vi "Clear.vi"(8 "error in (no error)":errorcluster, 11 "Execution UI In":refnum<class "Execution UI.lvclass">) -> (0 "error out":errorcluster)   [LabVIEW 2020, in "Execution UI.lvclass"]
uses:
  Execution UI.lvclass
  Execution UI.lvclass/Execution UI.ctl
  Process/Process.lvclass
  Result Model/Result Model.lvclass
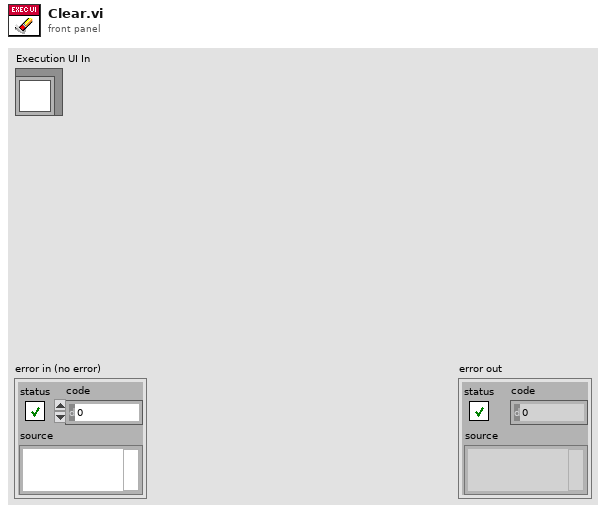
[diagram p1: front panel]
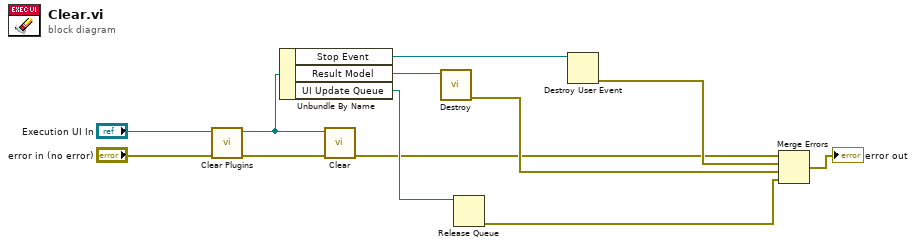
[diagram p0: block diagram]
diagram:
  n1 = call "Clear Plugins.vi"("error in (no error)"="error in (no error)", "Execution UI in"="Execution UI In") -> ("error out"=w2:errorcluster, "Execution UI out"=w3:refnum<class "Execution UI.lvclass">)  [unwired: 8 in]
  n2 = Unbundle By Name(w3) -> ("Stop Event"=w10:refnum<user-event>, "Result Model"=w8:refnum<class "Result Model.lvclass">, "UI Update Queue"=w6:refnum<queue>)
  n3 = call-parent "Clear.vi"("error in (no error)"=w2, "Process In"=w3) -> ("error out"=w1:errorcluster)  [unwired: 9 in]
  n4 = call "Destroy.vi"("Result Model in"=w8) -> ("error out"=w7:errorcluster)  [unwired: 10 in]
  n5 = Release Queue(queue=w6) -> (error out=w5:errorcluster)  [unwired: 2 in, 2 out]
  n6 = Destroy User Event(user event=w10) -> (error out=w9:errorcluster)  [unwired: 1 in]
  n7 = Merge Errors(w1, w9, w7, w5) -> (→"error out":errorcluster)
